vi "Caculate New MarkPoint.vi"(7 "DeltaM2-m1":cluster{"X":dbl, "Y":dbl}, 10 "Mark 2Vision":T1, 11 "Mark 1Vision":T1) -> (2 "New Mark 2Robot Point":cluster{dbl, dbl}, 3 "New Mark 1Robot Point":cluster{dbl, dbl})   [LabVIEW 2019]
uses:
  Function/UpVision/Ctrl/UpColorImg.ctl
  Function/UpVision/Ctrl/UpEnum_VisionCalibSet_Act.ctl
  LLB/Commonly VI/FilterPointNameToFloat.vi
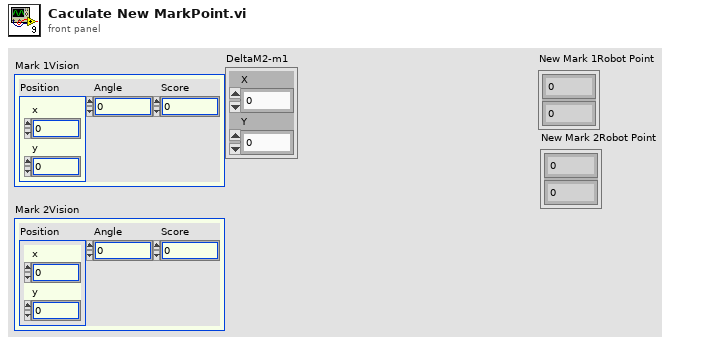
[diagram p1: front panel]
types:
  T1 = cluster{"Position":cluster{"x":sgl, "y":sgl}, "Angle":sgl, "Score":sgl}
  T2 = typedef "UpEnum_VisionCalibSet_Act.ctl" = enum16{"initial", "initialref", "save", "load", "UpDataToUI", "write", "read"}
  T3 = typedef "UpColorImg.ctl" = enum16{"CUpCam", "CUpSource", "CUpShow", "CUpToProcess1", "CUpToProcess2", "CUpForMatch", "CUpForCheckNumbers", "CupPreProcess"}
  T4 = enum16{"Initial", "Load", "Save", "Read", "WriteSpeed", "WritePoint"}
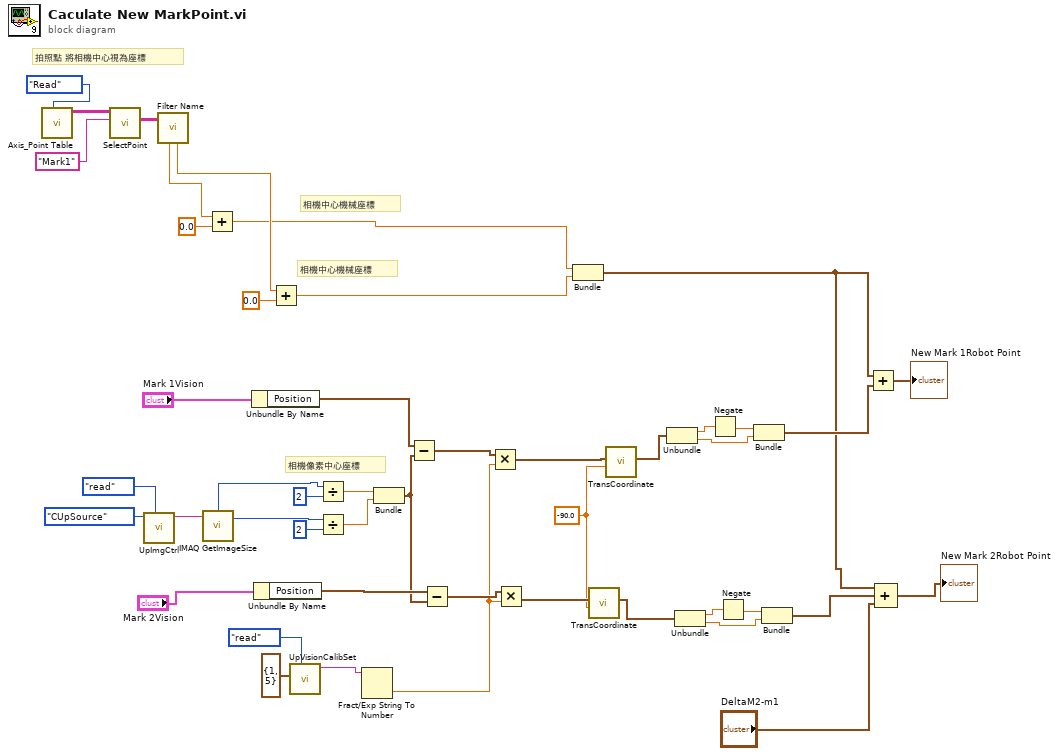
[diagram p0: block diagram]
diagram:
  w19 = sgl -90.0 ("A")
  # "相機像素中心座標"
  # "相機中心機械座標"
  # "相機中心機械座標"
  # "拍照點 將相機中心視為座標"
  n1 = call "Axis_Point Table.vi"("Enum"=T4."Read") -> ("RobotPoint"=w47:string[][])  [unwired: 8 in, 2 out]
  n2 = call "SelectPoint.vi"("PointName"="Mark1", "RobotPointsTableIn"=w47) -> ("RobotPointsOut"=w44:string[][])  [unwired: 7 in, 2 out]
  n3 = call "UpImgCtrl.vi"("Action"=enum16{"Initial", "read", "release"}."read", "ColorImg 2"=UpColorImg."CUpSource") -> ("ColorImg"=w39:string)  [unwired: 7 in, 2 out]
  n4 = call-poly "Filter Name.vi"("RobotPoints in"=w44) -> ("Y"=w42:dbl, "X"=w43:dbl)  [unwired: 4 in, 5 out]
  n5 = call "IMAQ GetImageSize"("Image"=w39) -> ("Y Resolution"=w35:i32, "X Resolution"=w38:i32)  [unwired: 3 in, 1 out]
  n6 = Add(x=w43, y=0.0) -> (x+y=w18:dbl)
  n7 = Unbundle By Name("Mark 1Vision") -> ("Position"=w31:cluster{"x":sgl, "y":sgl})
  n8 = Unbundle By Name("Mark 2Vision") -> ("Position"=w29:cluster{"x":sgl, "y":sgl})
  n9 = Add(x=w42, y=0.0) -> (x+y=w17:dbl)
  n10 = call "UpVisionCalibSet.vi"("Enum"=UpEnum_VisionCalibSet_Act."read", "indedx"=cluster{"Y":i32, "X":i32} {"Y"=1, "X"=5}) -> ("DataOut"=w24:string)  [unwired: 8 in, 1 out]
  n11 = Divide(x=w38, y=2) -> (x/y=w33:dbl)
  n12 = Divide(x=w35, y=2) -> (x/y=w32:dbl)
  n13 = Fract/Exp String To Number(string=w24) -> (number=w22:dbl)  [unwired: 3 in, 1 out]
  n14 = Bundle(w33, w32) -> (w28:cluster{dbl, dbl})  [unwired: 1 in]
  n15 = Subtract(x=w31, y=w28) -> (x-y=w27:cluster{dbl, dbl})
  n16 = Subtract(x=w29, y=w28) -> (x-y=w23:cluster{dbl, dbl})
  n17 = Multiply(x=w27, y=w22) -> (x*y=w21:cluster{dbl, dbl})
  n18 = Multiply(x=w23, y=w22) -> (x*y=w20:cluster{dbl, dbl})
  n19 = Bundle(w18, w17) -> (w2:cluster{dbl, dbl})  [unwired: 1 in]
  n20 = call "TransCoordinate.vi"("A"=w19, "Point in"=w20) -> ("Point out"=w4:cluster{"x":sgl, "y":sgl})  [unwired: 9 in]
  n21 = call "TransCoordinate.vi"("A"=w19, "Point in"=w21) -> ("Point out"=w12:cluster{"x":sgl, "y":sgl})  [unwired: 9 in]
  n22 = Unbundle(w12) -> ("x"=w11:sgl, "y"=w9:sgl)
  n23 = Unbundle(w4) -> ("x"=w5:sgl, "y"=w7:sgl)
  n24 = Negate(x=w11) -> (-x=w10:sgl)
  n25 = Negate(x=w5) -> (-x=w6:sgl)
  n26 = Bundle(w10, "y"=w9) -> (w8:cluster{sgl, "y":sgl})  [unwired: 1 in]
  n27 = Bundle(w6, "y"=w7) -> (w3:cluster{sgl, "y":sgl})  [unwired: 1 in]
  n28 = Add(x=w2, y=w8) -> (x+y=→"New Mark 1Robot Point":cluster{dbl, dbl})
  n29 = Compound Arithmetic op=ADD(w2, w3, "DeltaM2-m1") -> (→"New Mark 2Robot Point":cluster{dbl, dbl})
